vi "UTIL_OPEN and LOAD QUEUE v1_0_0.vi"(6 "Queue elements":string[](array[string])=["Initialize"], 7 "Flush queue first":bool, 8 "error in (no error)":errorcluster, 11 "Path":path) -> (0 "error out":errorcluster, 3 "Queue out":refnum<queue>)   [LabVIEW 2015]
doc: "UTIL_OPEN and LOAD QUEUE v1_0_0.vi\n\nCreates/Loads a queue by the name of the calling vi (minus the extension.vi). It then either flushes the items already on the queue then adds any additional Queue elements or just simply adds any new Queue elements to the queue and passes the queue reference out.\n\nCreated 2006 by\n\nJ. Daren Suntych\nNational Analytics\n970-397-0764"
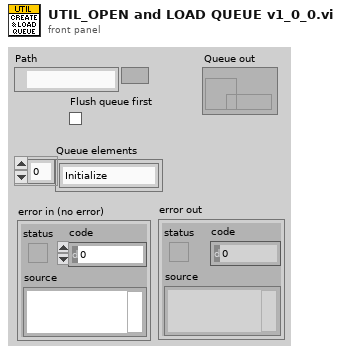
[diagram p1: front panel]
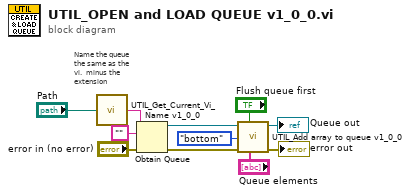
[diagram p0: block diagram]
diagram:
  # "Name the queue\nthe same as the\nvi.  minus the\nextension"
  n1 = call "UTIL_Get_Current_Vi_Name v1_0_0.vi"("Path"="Path") -> ("Name Minus Extention"=w9:string)  [unwired: 14 out]
  n2 = Obtain Queue(name (unnamed)=w9, element data type="", error in (no error)="error in (no error)") -> (queue out=w8:refnum<queue>, error out=w7:errorcluster)  [unwired: 2 in, 1 out]
  n3 = call "UTIL_Add array to queue v1_0_0.vi"("Queue elements"="Queue elements", "Flush (f)"="Flush queue first", "error in (no error)"=w7, "Queue position"=enum16{"top", "bottom"}."bottom", "Queue in"=w8) -> ("error out"=→"error out":errorcluster, "Queue out"=→"Queue out":refnum<queue>)  [unwired: 5 out]
